vi "Write_NetworkStram_OCU_Override.vi"(0 "VKey":T1, 1 "NetworkStreamWriter in":refnum<class "NetworkStreamWriter.lvclass">, 5 "Mainsail Position":T4, 7 "Jib Position":T3, 9 "Rudder Setpoint":T2 min=-1.0 max=1.0 scale=1.0..-1.0, 11 "error in (no error)":errorcluster, 12 "OverrideMode":T5) -> (3 "NetworkStreamWriter out":refnum<class "NetworkStreamWriter.lvclass">, 4 "Main Position":T4, 6 "Jib Position":T3, 8 "Rudder Position":T2 min=-1.0 max=1.0 scale=1.0..-1.0, 15 "error out":errorcluster)   [LabVIEW 2013]
doc: "Takes in the key value pressed and changes the value of the main sail, jib, and rudder accordingly with the following mapping of the arrow keys (ish):\n\n\"Page Up\" -- rudder right | \"Up\" -- Main out | \"Page Down\" -- Jib out\n\"Left\" -- rudder left | \"Down\" -- Main in | \"Right\" -- Jib in\n\nIt then bundles the main sail, jib sail, and rudder override commands and sends them to the boat using NetworkStreams. It also bundles with them the override mode so the Forebrain Sense can determine which actuator setting so implement and which to ignore. Deals with coersions, becaues humans can be silly.\n\n\n\nWritten by Victoria Coleman 04/12/14"
uses:
  cRIO_Code/Data/TypeDefs/Sail Set Suggestions.ctl
  cRIO_Code/Data/TypeDefs/OverrideMode.ctl
  cRIO_Code/Data/TypeDefs/MainsailPositionIndicator.ctl
  cRIO_Code/Data/TypeDefs/JibPositionIndicator.ctl
  cRIO_Code/Data/TypeDefs/Rudder Set Suggestions.ctl
  <vilib>/event_ctls.llb/eventvkey.ctl
  Writer/NetworkStreamWriter.lvclass
  cRIO_Code/Data/TypeDefs/OverrideInformation.ctl
  OCU/CommandMessages.ctl
panel:
  in  "Sail Suggesstions":T6 {"MainSailSuggestion" min=0.0 max=1.0; "JibSailSuggestion" min=0.0 max=1.0}
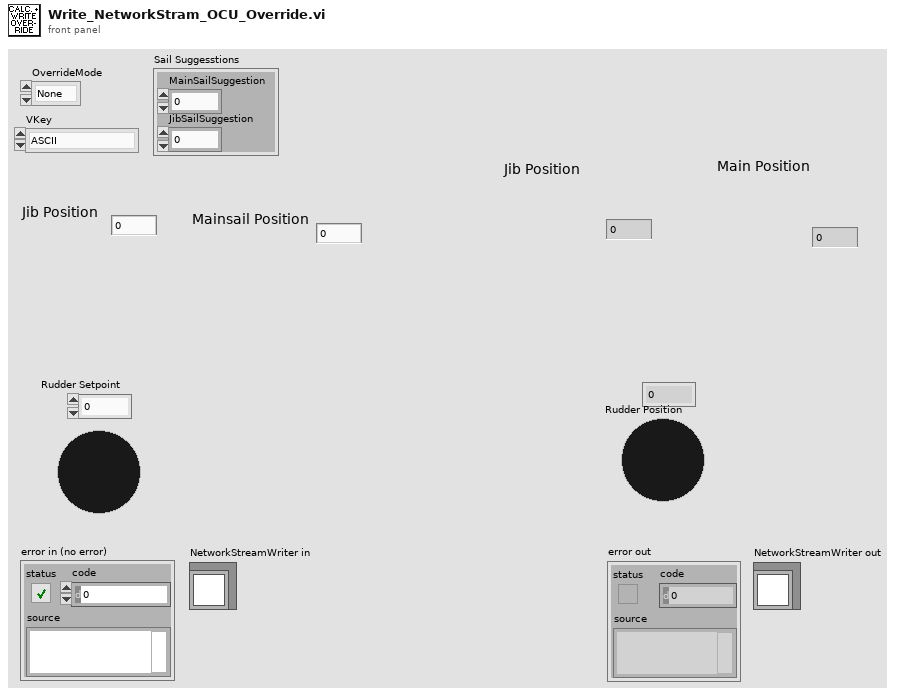
[diagram p1: front panel]
types:
  T1 = typedef "eventvkey.ctl" = enum16{"ASCII", "Enter", "Return", "Shift", "Ctrl", "Alt", "Cmd", "Opt", "Caps", "NumLock", "Clear", "Break", "Up", "Down", "Left", "Right", "Insert", "Delete", "Home", "End", "PageUp", "PageDown", "Escape", "Help", "Pause", "ScrollLock", "F1", "F2", "F3", "F4", "F5", "F6", "F7", "F8", "F9", "F10", "F11", "F12", "F13", "F14", "F15", "F16", "F17", "F18", "F19", "F20", "F21", "F22", "F23", "F24", "Play", "VolumeUp", "VolumeDown", "Mute", "Two Byte Char"}
  T2 = typedef "Rudder Set Suggestions.ctl" = dbl
  T3 = typedef "JibPositionIndicator.ctl" = dbl
  T4 = typedef "MainsailPositionIndicator.ctl" = dbl
  T5 = typedef "OverrideMode.ctl" = enum16{"None", "Rudder", "Sails", "Both"}
  T6 = typedef "Sail Set Suggestions.ctl" = cluster{"MainSailSuggestion":dbl, "JibSailSuggestion":dbl}
  T7 = typedef "CommandMessages.ctl" = enum16{"Boat Type", "Pass", "OverrideMode", "Add mission", "Delete mission", "Change constants"}
  T8 = typedef "OverrideInformation.ctl" = cluster{"OverrideMode":T5, "SailSetting":T6, "Rudder Setpoint":T2}
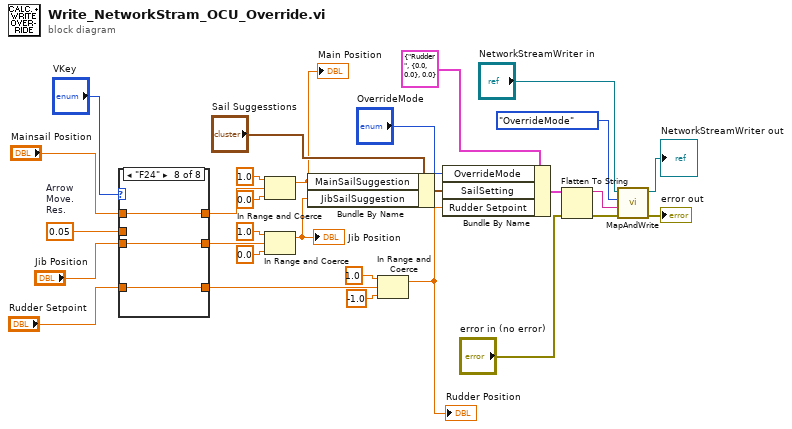
[diagram p0: block diagram]
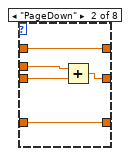
[diagram p3: hidden frame]
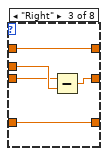
[diagram p4: hidden frame]
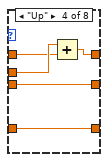
[diagram p5: hidden frame]
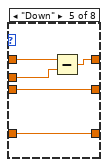
[diagram p6: hidden frame]
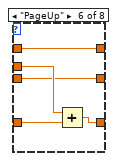
[diagram p7: hidden frame]
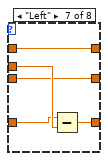
[diagram p8: hidden frame]
diagram:
  w24 = T4 0.05  # Arrow Move. Res.
  n1 = case shown="\"F24\"" "VKey" {
    tunnel: "Rudder Setpoint" -> [w30 w34 w40 w45 w49 w56 w61 w63]
    tunnel: "Jib Position" -> [w31 w36 w39 w43 w50 w55 w60 w64]
    tunnel: "Mainsail Position" -> [w32 w35 w38 w46 w52 w54 w59 w65]
    tunnel: w24 -> [_ w37 w42 w47 w51 w57 w62 _]
    tunnel: [w31 w33 w41 w43 w50 w55 w60 w64] -> w28
    tunnel: [w32 w35 w38 w44 w48 w54 w59 w65] -> w22
    tunnel: [w30 w34 w40 w45 w49 w53 w58 w63] -> w12
    frame "ASCII", Default {
    }
    frame "PageDown" {
      n2 = Add(x=w37, y=w36) -> (x+y=w33:T4)
    }
    frame "Right" {
      n3 = Subtract(x=w39, y=w42) -> (x-y=w41:T3)
    }
    frame "Up" {
      n4 = Add(x=w47, y=w46) -> (x+y=w44:T4)
    }
    frame "Down" {
      n5 = Subtract(x=w52, y=w51) -> (x-y=w48:T4)
    }
    frame "PageUp" {
      n6 = Add(x=w57, y=w56) -> (x+y=w53:T4)
    }
    frame "Left" {
      n7 = Subtract(x=w61, y=w62) -> (x-y=w58:T2)
    }
    frame "F24" {
    }
  }
  n8 = In Range and Coerce(upper limit=T4 1.0, x=w22, lower limit=T4 0.0) -> (coerced(x)=w14:T4)  [unwired: 1 out]
  "Main Position" <- w14
  n9 = In Range and Coerce(upper limit=T3 1.0, x=w28, lower limit=T3 0.0) -> (coerced(x)=w15:T3)  [unwired: 1 out]
  "Jib Position" <- w15
  n10 = Bundle By Name(cluster="Sail Suggesstions", "MainSailSuggestion"=w14, "JibSailSuggestion"=w15) -> (w20:T6)
  n11 = In Range and Coerce(upper limit=T2 1.0, x=w12, lower limit=T2 -1.0) -> (coerced(x)=w11:T2)  [unwired: 1 out]
  "Rudder Position" <- w11
  n12 = Bundle By Name(cluster=T8 {"OverrideMode"=enum."Rudder", "SailSetting"={"MainSailSuggestion"=0.0, "JibSailSuggestion"=0.0}, "Rudder Setpoint"=0.0} ("OverrideInfo"), "OverrideMode"="OverrideMode", "SailSetting"=w20, "Rudder Setpoint"=w11) -> (w19:T8)
  n13 = Flatten To String(anything=w19, error in (no error)="error in (no error)") -> (data string=w17:string, error out=w18:errorcluster)  [unwired: 2 in, 1 out]
  n14 = call "MapAndWrite.vi"("error in (no error)"=w18, "String_Cast_of_Info"=w17, "Commands"=CommandMessages."OverrideMode", "NetworkStreamWriter in"="NetworkStreamWriter in") -> ("error out"=→"error out":errorcluster, "NetworkStreamWriter out"=→"NetworkStreamWriter out":refnum<class "NetworkStreamWriter.lvclass">)  [unwired: 2 in]
